vi "Teleop_Calc_Fly_L.vi"(11 "Teleop Local Data in":T1) -> (3 "Teleop Local Data out":T1)   [LabVIEW 2016]
uses:
  Typedefs/typedef_cluster_Teleop Local Data.ctl
  Typedefs/typedef_enum_Joystick Buttons.ctl
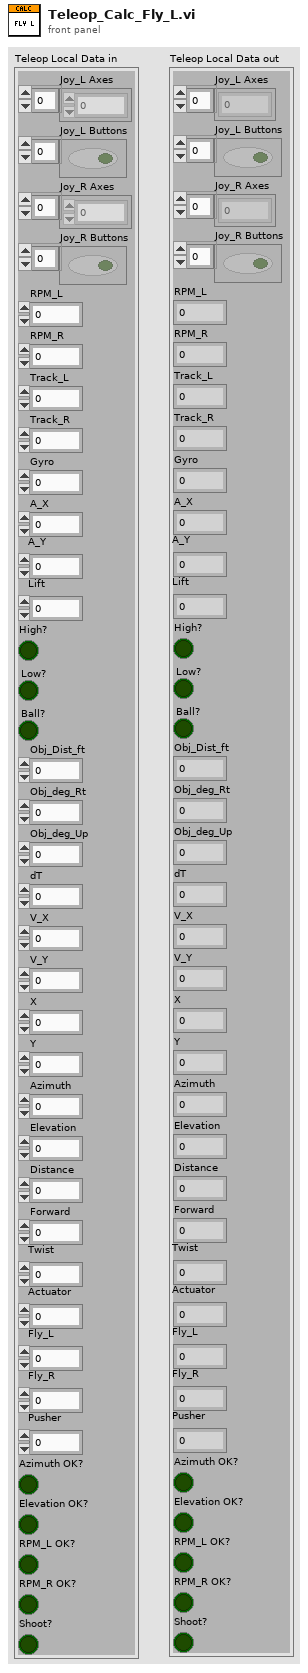
[diagram p1: front panel]
types:
  T1 = typedef "typedef_cluster_Teleop Local Data.ctl" = cluster{"Joy_L Axes":dbl[], "Joy_L Buttons":bool[], "Joy_R Axes":dbl[], "Joy_R Buttons":bool[], "RPM_L":dbl, "RPM_R":dbl, "Track_L":dbl, "Track_R":dbl, "Gyro":dbl, "A_X":dbl, "A_Y":dbl, "Lift":dbl, "High?":bool, "Low?":bool, "Ball?":bool, "Obj_Dist_ft":dbl, "Obj_deg_Rt":dbl, "Obj_deg_Up":dbl, "dT":dbl, "V_X":dbl, "V_Y":dbl, "X":dbl, "Y":dbl, "Azimuth":dbl, "Elevation":dbl, "Distance":dbl, "Forward":dbl, "Twist":dbl, "Actuator":dbl, "Fly_L":dbl, "Fly_R":dbl, "Pusher":dbl, "Azimuth OK?":bool, "Elevation OK?":bool, "RPM_L OK?":bool, "RPM_R OK?":bool, "Shoot?":bool}
  T2 = typedef "typedef_enum_Joystick Buttons.ctl" = enum16{"Trigger", "Thumb", "Top3", "Top4", "Top5", "Top6", "Low7", "Low8", "Low9", "Low10", "Low11", "Low12", "Hat0", "Hat1", "Hat2", "Hat3", "Hat4", "Hat5", "Hat6", "Hat7", "Hat8"}
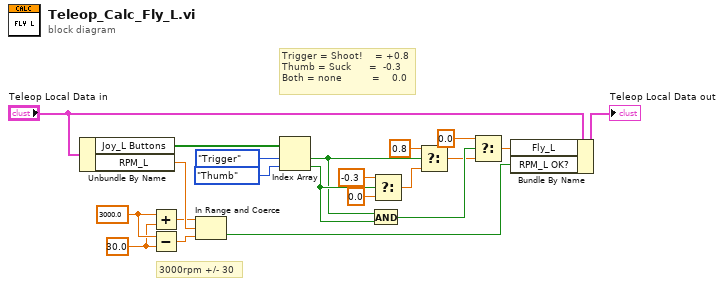
[diagram p0: block diagram]
diagram:
  w14 = 30.0 ("upper limit")
  w15 = 3000.0 ("upper limit")
  # "Trigger = Shoot!    = +0.8\nThumb = Suck      =  -0.3\nBoth = none          =    0.0"
  # "3000rpm +/- 30"
  n1 = Unbundle By Name("Teleop Local Data in") -> ("Joy_L Buttons"=w18:bool[], "RPM_L"=w16:dbl)
  n2 = Add(x=w15, y=w14) -> (x+y=w13:dbl)
  n3 = Subtract(x=w15, y=w14) -> (x-y=w12:dbl)
  n4 = In Range and Coerce(upper limit=w13, x=w16, lower limit=w12) -> (In Range?=w11:bool)  [unwired: 1 out]
  n5 = Index Array(array=w18, index #1=typedef_enum_Joystick_Buttons."Trigger" ("Joystick Buttons"), index #2=typedef_enum_Joystick_Buttons."Thumb" ("Joystick Buttons")) -> (element #1=w5:bool, element #2=w6:bool)
  n6 = And(x=w5, y=w6) -> (x .and. y?=w4:bool)
  n7 = Select(t=-0.3, s=w6, f=0.0) -> (s? t:f=w8:dbl)
  n8 = Select(t=0.8, s=w5, f=w8) -> (s? t:f=w3:dbl)
  n9 = Select(t=0.0, s=w4, f=w3) -> (s? t:f=w2:dbl)
  n10 = Bundle By Name(cluster="Teleop Local Data in", "Fly_L"=w2, "RPM_L OK?"=w11) -> (→"Teleop Local Data out":T1)
